vi "Set_Joint_Main_Loop_EMG_Control.vi"(0 "X-CAN in":refnum<class "X-CAN.lvclass">, 1 "Actual position":T2(array[cluster]) {"Error Code" format="%b"; "ID" format="%x"}, 2 "Motor enabled?":bool, 5 "Reset?":bool[](array[boolean]), 7 "EMG control":T1(ring), 9 "Current position":u16[](array[numeric]) format="%x", 11 "error in (no error)":errorcluster, 12 "Speed":u16[](array[numeric]) format="%x") -> (4 "X-CAN out":refnum<class "X-CAN.lvclass">, 6 "New position":T2(array[cluster]) {"Error Code" format="%b"; "ID" format="%x"}, 15 "error out":errorcluster)   [LabVIEW 2015]
uses:
  <vilib>/Stratom, Inc/X-CAN for myRIO (API)/X-CAN Class/X-CAN.lvclass
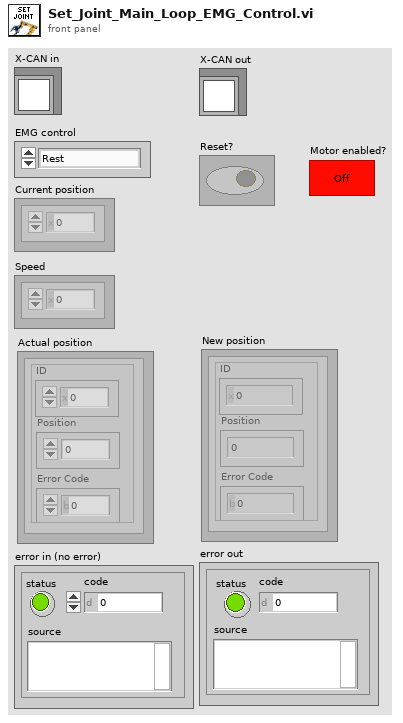
[diagram p1: front panel]
types:
  T1 = enum16{"Rest", "Biceps contracted", "Triceps contracted"}
  T2 = cluster{"ID":u8, "Position":u16, "Error Code":u8}[]
  T3 = typedef "X-CAN.lvclass/CANFrame.ctl" = cluster{"identifier":u32, "extended?":bool, "echo?":bool, "payload":u8[], "timestamp":timestamp}
  T4 = cluster{"Error Code":u8, "Position":u16, "ID":u8}
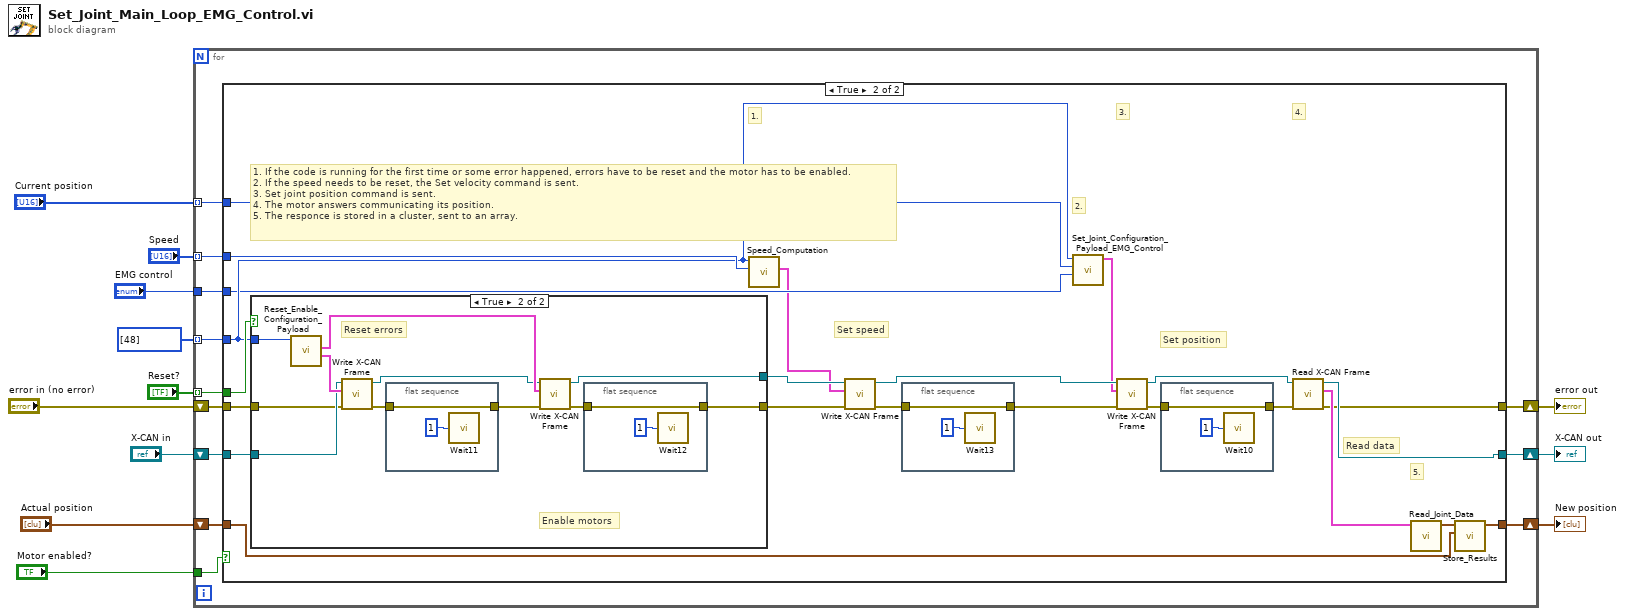
[diagram p0: block diagram]
diagram:
  n1 = for {
    shift-right: [w19] -> w9
    shift-left: "X-CAN in" -> [w24]
    shift-right: [w15] -> w10
    shift-left: "error in (no error)" -> [w23]
    tunnel: u8[] [48] ("identifier") -> [w17] mode=indexing
    tunnel: "Reset?" -> [w22] mode=indexing
    tunnel: "Current position" -> [w18] mode=indexing
    shift-right: [w21] -> w4
    shift-left: "Actual position" -> [w20]
    tunnel: "Speed" -> [w16] mode=indexing
    tunnel: "Motor enabled?" -> [w14]
    tunnel: "EMG control" -> [w13]
    n2 = case shown="True" w14 {
      tunnel: w24 -> [w26 w49]
      tunnel: w23 -> [w27 w48]
      tunnel: w22 -> [_ w47]
      tunnel: [w25 w46] -> w21
      tunnel: w20 -> [w25 w45]
      tunnel: [w26 w41] -> w19
      tunnel: w18 -> [_ w31]
      tunnel: w13 -> [_ w30]
      tunnel: w17 -> [_ w32]
      tunnel: w16 -> [_ w39]
      tunnel: [w27 w34] -> w15
      frame False {
      }
      frame True {
        # "Set speed"
        # "1. If the code is running for the first time or some error happened, errors have to be reset and the motor has to be enabled.\n2. If the speed needs to be reset, the Set velocity command is sent.\n3. Set joint position command is sent.\n4. The motor answers communicating its position.\n5. The responce is stored in a cluster, sent to an array."
        # "5."
        # "4."
        # "3."
        # "2."
        # "1."
        # "Read data"
        # "Set position"
        n3 = case shown="True" w47 {
          tunnel: [w54 w59] -> w38
          tunnel: [w53 w58] -> w37
          tunnel: w49 -> [w54 w57]
          tunnel: w48 -> [w53 w56]
          tunnel: w32 -> [_ w55]
          frame False {
          }
          frame True {
            # "Enable motors"
            # "Reset errors"
            n4 = call "Reset_Enable_Configuration_Payload.vi"("identifier selection in"=w55) -> ("Reset errors command"=w61:T3, "Enable motor command"=w62:T3)  [unwired: 9 in]
            n5 = call <vilib>:"Write X-CAN Frame.vi"("error in"=w56, "CAN Frame"=w61, "X-CAN Session in"=w57) -> ("error out"=w63:errorcluster, "X-CAN Session out"=w60:refnum<class "X-CAN.lvclass">)  [unwired: 7 in]
            n6 = flat-sequence {
              tunnel: w63 -> [w68]
              tunnel: [w68] -> w65
              frame #0 {
                n7 = call "Wait11"("Count(mSec)"=u32 1 ("Tick Count(mSec)")) -> ()  [unwired: 1 out]
              }
            }
            n8 = call <vilib>:"Write X-CAN Frame.vi"("error in"=w65, "CAN Frame"=w62, "X-CAN Session in"=w60) -> ("error out"=w64:errorcluster, "X-CAN Session out"=w59:refnum<class "X-CAN.lvclass">)  [unwired: 7 in]
            n9 = flat-sequence {
              tunnel: w64 -> [w66]
              tunnel: [w66] -> w58
              frame #0 {
                n10 = call "Wait12"("Count(mSec)"=u32 1 ("Tick Count(mSec)")) -> ()  [unwired: 1 out]
              }
            }
          }
        }
        n11 = call "Speed_Computation.vi"("Speed"=w39, "identifier"=w32) -> ("output cluster"=w29:T3)  [unwired: 9 in]
        n12 = call <vilib>:"Write X-CAN Frame.vi"("error in"=w37, "CAN Frame"=w29, "X-CAN Session in"=w38) -> ("error out"=w28:errorcluster, "X-CAN Session out"=w36:refnum<class "X-CAN.lvclass">)  [unwired: 7 in]
        n13 = flat-sequence {
          tunnel: w28 -> [w51]
          tunnel: [w51] -> w35
          frame #0 {
            n14 = call "Wait13"("Count(mSec)"=u32 1 ("milliseconds to wait")) -> ()  [unwired: 1 out]
          }
        }
        n15 = call "Set_Joint_Configuration_Payload_EMG_Control.vi"("EMG control"=w30, "Current position"=w31, "Identifier selection in"=w32) -> ("Set joint position command"=w33:T3)  [unwired: 8 in]
        n16 = call <vilib>:"Write X-CAN Frame.vi"("error in"=w35, "CAN Frame"=w33, "X-CAN Session in"=w36) -> ("error out"=w50:errorcluster, "X-CAN Session out"=w43:refnum<class "X-CAN.lvclass">)  [unwired: 7 in]
        n17 = flat-sequence {
          tunnel: w50 -> [w70]
          tunnel: [w70] -> w42
          frame #0 {
            n18 = call "Wait10"("Count(mSec)"=u32 1 ("milliseconds to wait")) -> ()  [unwired: 1 out]
          }
        }
        n19 = call <vilib>:"Read X-CAN Frame.vi"("error in"=w42, "X-CAN Session in"=w43) -> ("error out"=w34:errorcluster, "CAN Frame"=w40:T3, "X-CAN Session out"=w41:refnum<class "X-CAN.lvclass">)  [unwired: 7 in]
        n20 = call "Read_Joint_Data.vi"("CAN Frame"=w40) -> ("Joint Position out"=w44:T4)  [unwired: 9 in, 1 out]
        n21 = call "Store_Results.vi"("Positions in"=w45, "Joint Info"=w44) -> ("Stored positions"=w46:T2)  [unwired: 9 in]
      }
    }
  }
  "error out" <- w10
  "X-CAN out" <- w9
  "New position" <- w4
